vi "Configure OSC CURRent OFFSet.vi"(6 "Range":u16=1 min=1 max=3 step=1, 8 "error in (no error)":errorcluster, 9 "Offset value":dbl=5e-07 min=0.0 max=5e-07 step=1e-12 format="%.3p", 10 "Step":u16=1 min=1 max=99 step=1, 11 "VISA resource in":refnum<visa-resource-name>) -> (0 "error out":errorcluster, 3 "VISA resource out":refnum<visa-resource-name>)   [LabVIEW 2025]
doc: "This VI set the OPEN limit for Open/Short Circuit (OSC) test mode.\nRange: 0.1 to 1, step 0.1"
uses:
  <instrlib>/Chroma 19052/Chroma 19052.lvlib
panel:
  # "Set OSC CURRENT OFFSET"
  # "[F]"
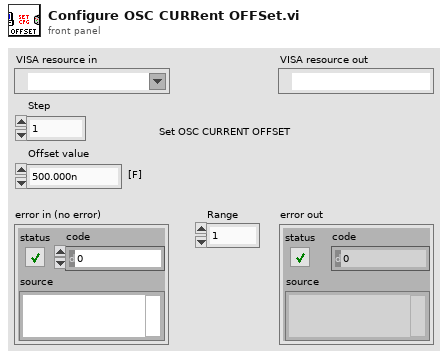
[diagram p1: front panel]
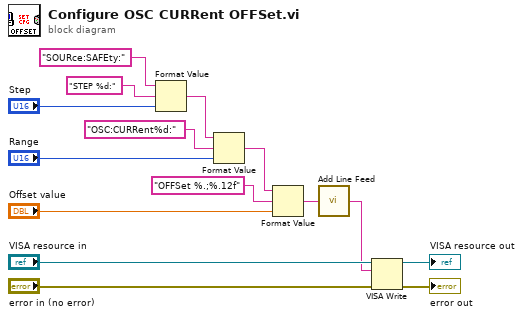
[diagram p0: block diagram]
diagram:
  n1 = Format Value(string ("")="SOURce:SAFEty:", format string="STEP %d:", value (0)="Step") -> (output string=w4:string)
  n2 = Format Value(string ("")=w4, format string="OSC:CURRent%d:", value (0)="Range") -> (output string=w2:string)
  n3 = Format Value(string ("")=w2, format string="OFFSet %.;%.12f", value (0)="Offset value") -> (output string=w1:string)
  n4 = call <instrlib>:"Add Line Feed.vi"("Command string"=w1) -> ("Concatenated string"=w9:string)  [unwired: 4 in]
  n5 = VISA Write(VISA resource name="VISA resource in", write buffer=w9, error in (no error)="error in (no error)") -> (VISA resource name out=→"VISA resource out":refnum<visa-resource-name>, error out=→"error out":errorcluster)  [unwired: 1 out]
